vi "Get Internal Counter Out Terminal.vi"(8 "error in (no error)":errorcluster, 11 "task in":refnum<k21>) -> (0 "error out":errorcluster, 2 "internal counter out":string, 3 "task out":refnum<k21>)   [LabVIEW 2013]
uses:
  <resource>/objmgr/daqmx.rc
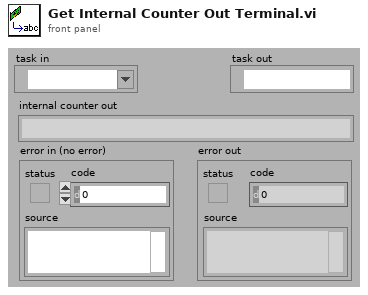
[diagram p1: front panel]
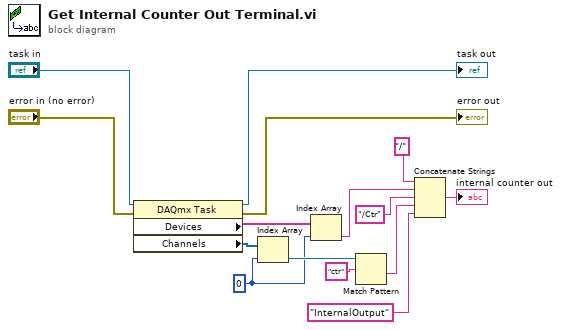
[diagram p0: block diagram]
diagram:
  w1 = 0 ("index")
  n1 = property class="DAQmx Task"(reference="task in", error in="error in (no error)") -> (reference out=→"task out":refnum<k21>, error out=→"error out":errorcluster, "Devices"=w7:tag[], "Channels"=w14:refnum<k21>[])
  n2 = Index Array(array=w14, index=w1) -> (element=w15:refnum<k21>)
  n3 = Index Array(array=w7, index=w1) -> (element=w9:tag)
  n4 = Match Pattern(string=w15, regular expression="ctr") -> (after substring=w11:string)  [unwired: 4 out]
  n5 = Concatenate Strings("/" ("string"), w9, "/Ctr" ("string"), w11, "InternalOutput" ("string")) -> (→"internal counter out":string)
